vi "CameraTuning.vi"(0 "Table VRN IN":refnum<visa-resource-name>="COM9", 2 "Table_Astrom":T1 {"CRVAL" format="%.6g"; "CD" format="%_7g"}, 7 "Offset":dbl min=0.0 max=5.0 step=0.25 format="%.2f", 11 "error IN":errorcluster) -> (3 "VIpath":path=path "C:/UdeM/OMM/Bonnette/Programme/BonOMM 7.1/VIs 7.1/CameraTuning.vi", 4 "Table VRN OUT":refnum<visa-resource-name>="COM9", 8 "Sortie_usager?":bool, 15 "error OUT":errorcluster)   [LabVIEW 2011]
uses:
  Globals.vi
panel:
  in  "Call for path ?":bool
  in  "Exit":bool
  in  "TiltBoxE":bool
  in  "TiltBoxO":bool
  in  "TiltBoxS":bool
  in  "TiltBoxN":bool
  # "La direction choisie sera\nappliquée au télescope."
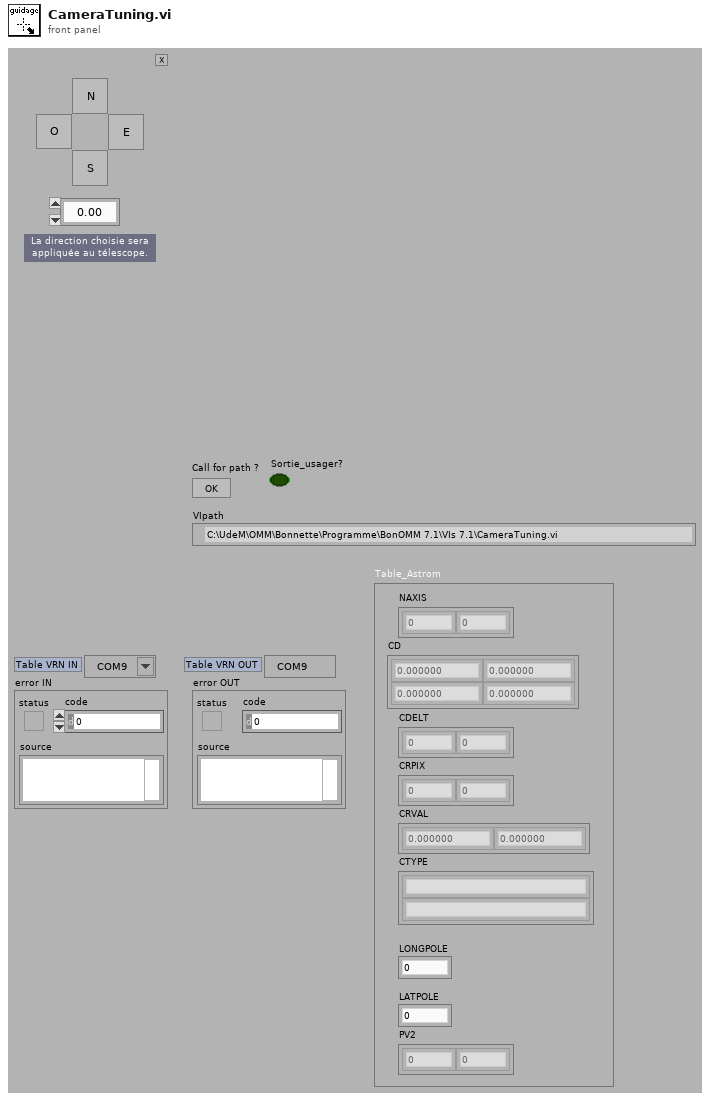
[diagram p1: front panel]
types:
  T1 = cluster{"NAXIS":dbl[], "CD":dbl[][], "CDELT":dbl[], "CRPIX":dbl[], "CTYPE":string[], "CRVAL":dbl[], "LONGPOLE":dbl, "LATPOLE":dbl, "PV2":dbl[]}
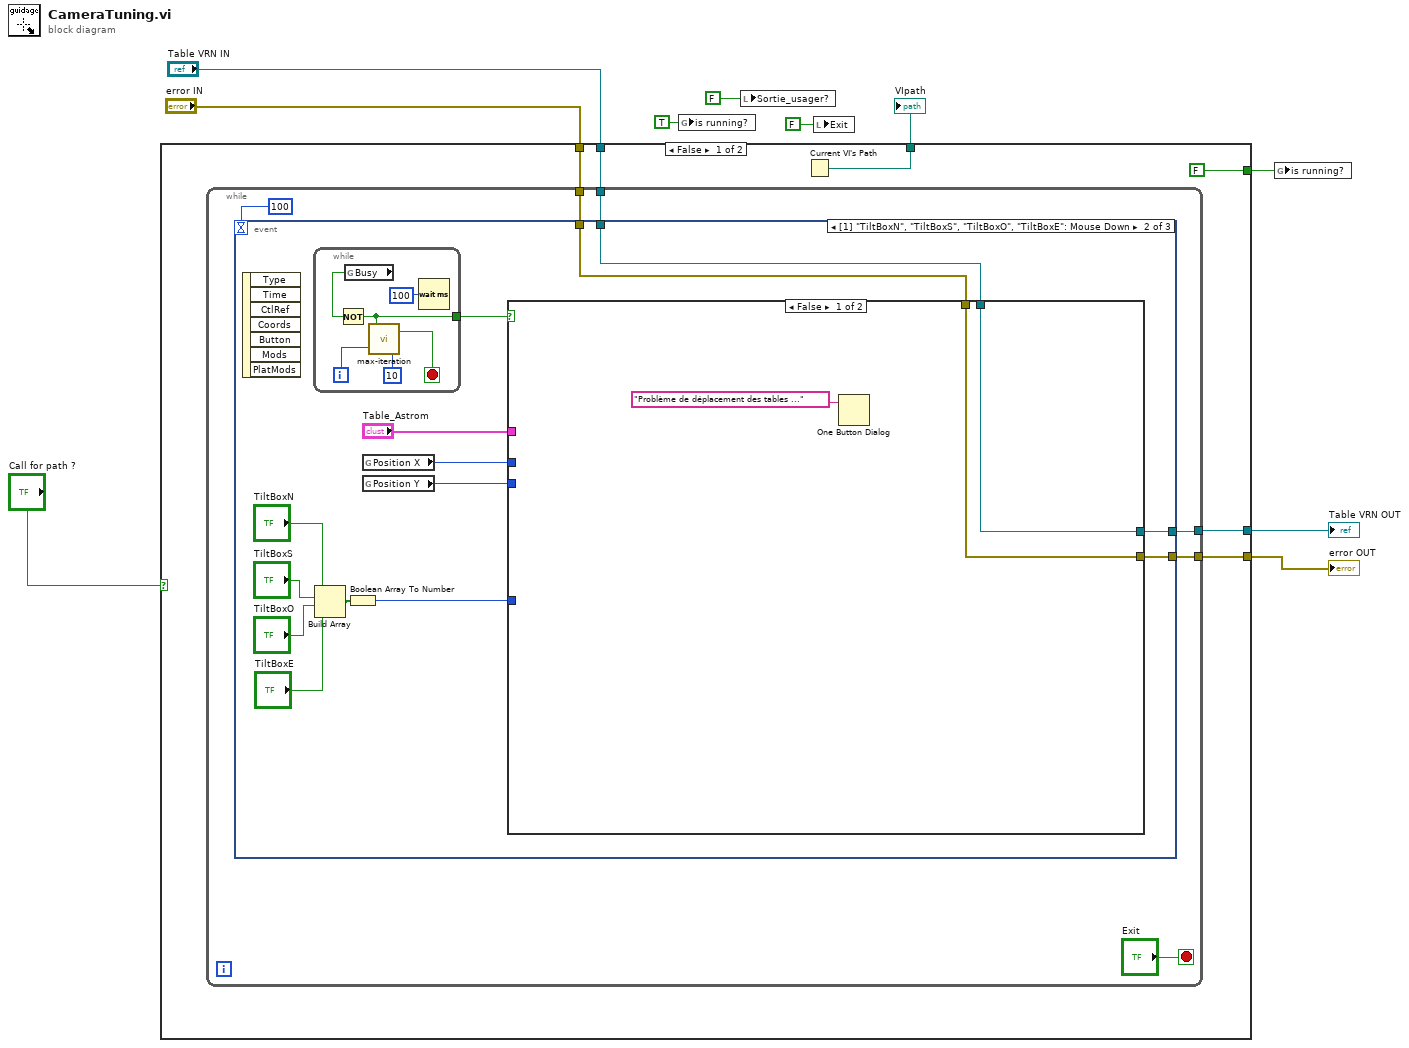
[diagram p0: block diagram]
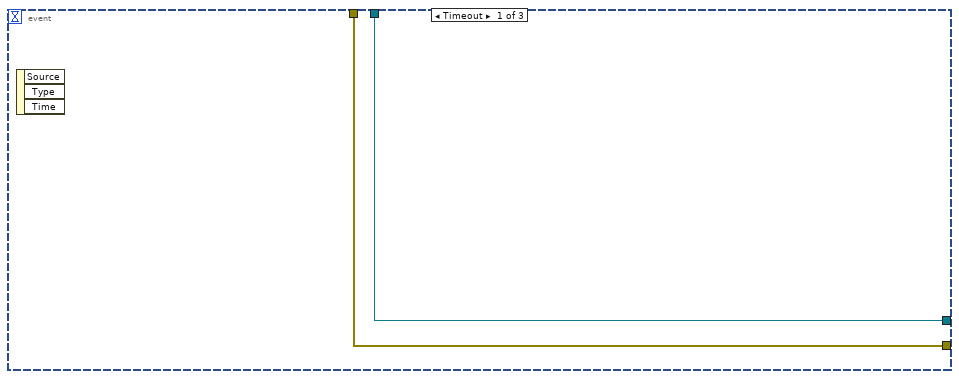
[diagram p2: hidden frame]
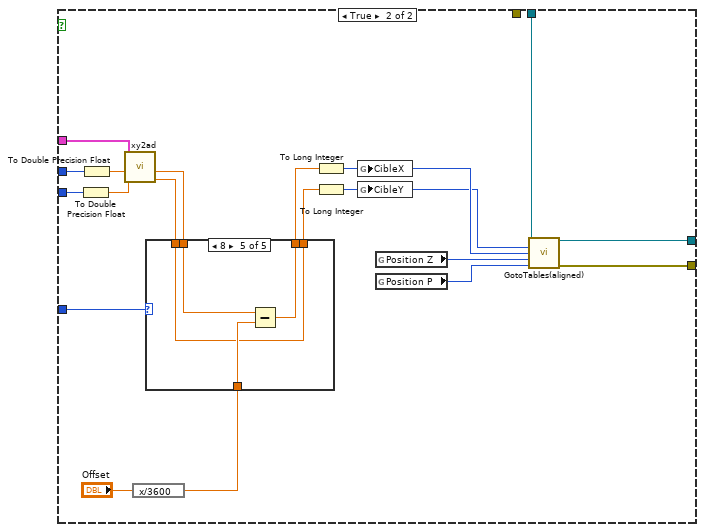
[diagram p3: hidden frame]
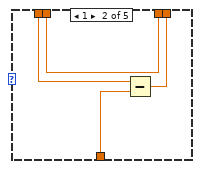
[diagram p5: hidden frame]
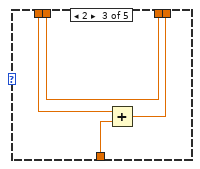
[diagram p6: hidden frame]
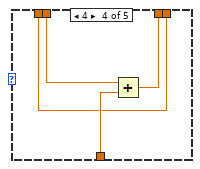
[diagram p7: hidden frame]
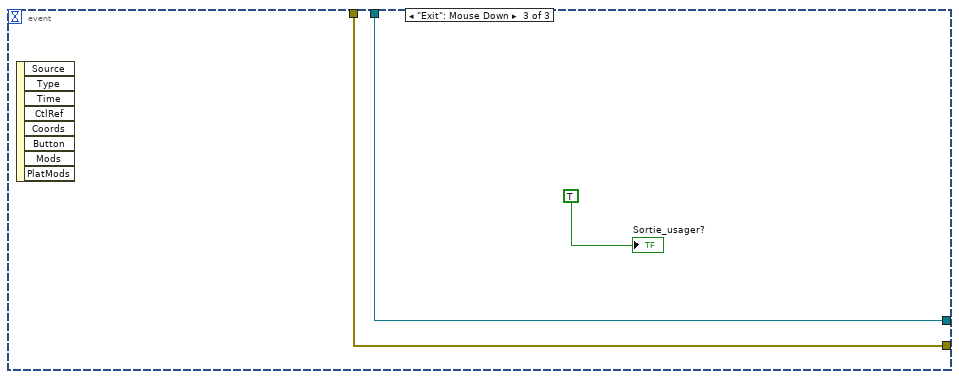
[diagram p8: hidden frame]
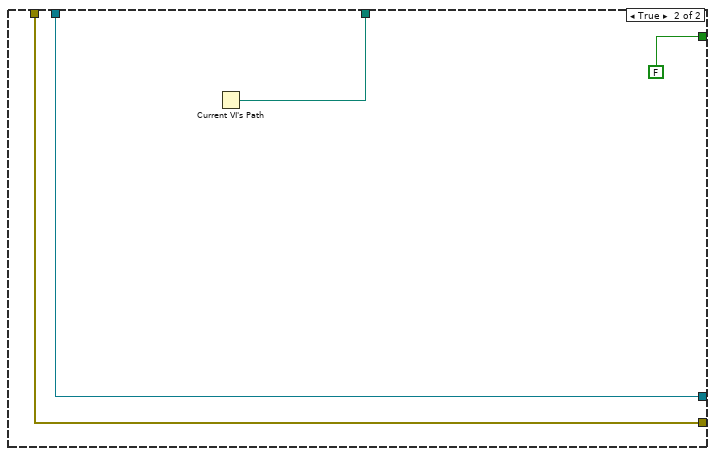
[diagram p9: hidden frame]
diagram:
  n1 = case shown="False" "Call for path ?" {
    tunnel: [w16 w91] -> w8
    tunnel: [FALSE ("Exit") FALSE ("Exit")] -> w6
    tunnel: "Table VRN IN" -> [w14 w89]
    tunnel: [w13 w89] -> w3
    tunnel: [w12 w88] -> w2
    tunnel: "error IN" -> [w11 w88]
    frame False {
      n2 = while {
        tunnel: [w20] -> w13
        tunnel: w14 -> [w19]
        tunnel: [w18] -> w12
        tunnel: w11 -> [w17]
        stop <- "Exit" stop-if-true
        n3 = event shown="[1] \"TiltBoxN\", \"TiltBoxS\", \"TiltBoxO\", \"TiltBoxE\": Mouse Down" {
          selector: _ -> [_ _ _]
          dyn-events: _ -> [_ _ _]
          timeout: 100 -> [_ _ _]
          tunnel: [w24 w28 w86] -> w20
          tunnel: w19 -> [w24 w27 w86]
          tunnel: [w23 w26 w85] -> w18
          tunnel: w17 -> [w23 w25 w85]
          event Timeout {
            n4 = event-data() -> ()  [unwired: 1 in, 3 out]
          }
          event "TiltBoxN", "TiltBoxS", "TiltBoxO", "TiltBoxE": Mouse Down {
            n5 = event-data() -> ()  [unwired: 1 in, 7 out]
            n6 = while {
              tunnel: [w79] -> w32
              i -> [w83]
              stop <- w84 stop-if-true
              n7 = global read "Globals.vi" "Busy"() -> (w80:bool)
              n8 = Not(x=w80) -> (.not. x?=w79:bool)
              n9 = call "max-iteration.vi"("i max"=10, "i act"=w83, "Valeur entrante"=w79) -> ("break ?"=w84:bool)
              n10 = Wait (ms)(milliseconds to wait=u32 100) -> ()  [unwired: 1 out]
            }
            n11 = Build Array("TiltBoxN", "TiltBoxS", "TiltBoxO", "TiltBoxE") -> (w34:bool[])
            n12 = Boolean Array To Number(Boolean array=w34) -> (number=w33:u32)
            n13 = global read "Globals.vi" "Position X"() -> (w29:i32)
            n14 = global read "Globals.vi" "Position Y"() -> (w30:i32)
            n15 = case shown="False" w32 {
              tunnel: w33 -> [_ w54]
              tunnel: w27 -> [w40 w48]
              tunnel: "Table_Astrom" -> [_ w60]
              tunnel: w30 -> [_ w59]
              tunnel: w29 -> [_ w58]
              tunnel: [w40 w43] -> w28
              tunnel: [w39 w42] -> w26
              tunnel: w25 -> [w39 _]
              frame False {
                n16 = One Button Dialog(message="Problème de déplacement des tables ...") -> ()  [unwired: 1 in, 1 out]
              }
              frame True {
                n17 = To Double Precision Float(number=w59) -> (double precision float=w56:dbl)
                n18 = To Double Precision Float(number=w58) -> (double precision float=w57:dbl)
                n19 = call "xy2ad.vi"("Y (px)"=w56, "X (px)"=w57, "Astrometry"=w60) -> ("DEC (°)"=w52:dbl, "RA (°)"=w53:dbl)  [unwired: 5 in, 2 out]
                n20 = expression code="x/3600"("Offset") -> (w51:dbl)
                n21 = case shown="8" w54 {
                  tunnel: w53 -> [w62 w63 w67 w73 w77]
                  tunnel: w52 -> [w61 w65 w69 w71 w75]
                  tunnel: w51 -> [_ w66 w70 w74 w78]
                  tunnel: [w62 w63 w67 w72 w76] -> w50
                  tunnel: [w61 w64 w68 w71 w75] -> w49
                  frame 0, Default {
                  }
                  frame 1 {
                    n22 = Subtract(x=w65, y=w66) -> (x-y=w64:dbl)
                  }
                  frame 2 {
                    n23 = Add(x=w69, y=w70) -> (x+y=w68:dbl)
                  }
                  frame 4 {
                    n24 = Add(x=w73, y=w74) -> (x+y=w72:dbl)
                  }
                  frame 8 {
                    n25 = Subtract(x=w77, y=w78) -> (x-y=w76:dbl)
                  }
                }
                n26 = To Long Integer(number=w50) -> (32bit integer=w47:i32)
                n27 = To Long Integer(number=w49) -> (32bit integer=w46:i32)
                n28 = global write "Globals.vi" "CibleX"(w47) -> ()
                n29 = global write "Globals.vi" "CibleY"(w46) -> ()
                n30 = global read "Globals.vi" "Position Z"() -> (w45:i32)
                n31 = global read "Globals.vi" "Position P"() -> (w44:i32)
                n32 = call "GotoTables(aligned).vi"("VRN IN"=w48, "Pulse Y"=w46, "Pulse X"=w47, "Pulse Z"=w45, "Pulse P"=w44) -> ("VRN OUT"=w43:refnum<visa-resource-name>, "error OUT"=w42:errorcluster)  [unwired: 8 in, 1 out]
              }
            }
          }
          event "Exit": Mouse Down {
            n33 = event-data() -> ()  [unwired: 1 in, 8 out]
            "Sortie_usager?" <- TRUE ("Exit")
          }
        }
      }
      n34 = Current VI's Path() -> (path=w16:path)
    }
    frame True {
      n35 = Current VI's Path() -> (path=w91:path)
    }
  }
  "VIpath" <- w8
  "Table VRN OUT" <- w3
  "error OUT" <- w2
  n36 = global write "Globals.vi" "is running?"(TRUE ("Exit")) -> ()
  n37 = local write "Sortie_usager?"(FALSE ("Exit")) -> ()
  n38 = local write "Exit"(FALSE ("Exit")) -> ()
  n39 = global write "Globals.vi" "is running?"(w6) -> ()
